vi "DAC.vi"(9 "编码位数L":dbl=8.0, 10 "量化阶Δ(V)":dbl=0.02, 11 "编码信号数组":digitalwaveform(waveform)) -> (3 "还原信号数组":dbl[](array[numeric]))   [LabVIEW 2018]
uses:
  <vilib>/Waveform/DWDTOps.llb/DWDT Digital to Binary U32.vi
panel:
  # "输入：编码信号数组（数字数据），量化阶Δ，编码位数L(=8)\n输出：还原信号数组（数组）"
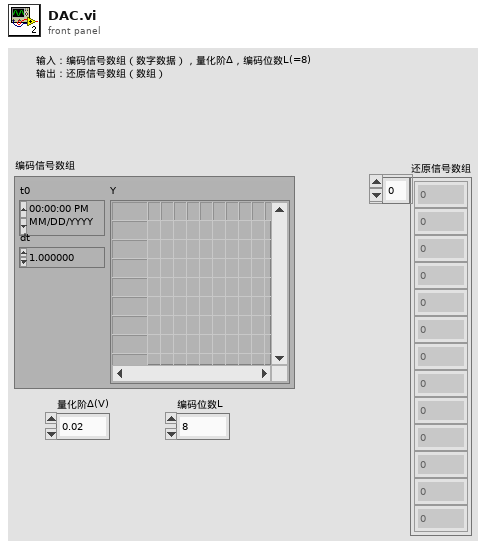
[diagram p1: front panel]
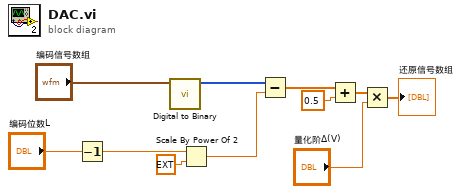
[diagram p0: block diagram]
diagram:
  n1 = Decrement(x="编码位数L") -> (x-1=w9:dbl)
  n2 = call-poly <vilib>:"Digital to Binary.vi"("digital waveform"="编码信号数组") -> ("binary array"=w7:u32[])  [unwired: 9 in, 1 out]
  n3 = Scale By Power Of 2(n=w9, x=ext 1.0) -> (x*2^n=w6:ext)
  n4 = Subtract(x=w7, y=w6) -> (x-y=w4:ext[])
  n5 = Add(x=w4, y=0.5) -> (x+y=w2:ext[])
  n6 = Multiply(x=w2, y="量化阶Δ(V)") -> (x*y=→"还原信号数组":ext[])
